vi "Dispose.vi"(8 "error in (no error)":errorcluster, 11 "BombedMazeGame":refnum<class "BombedMazeGame.lvclass">) -> (0 "error out":errorcluster)   [LabVIEW 2020, in "FactoryMethod.lvlib" / "NoParametrizedFactoryMethod.lvlib" / "BombedMazeGame.lvclass"]
uses:
  BombedMazeGame.lvclass
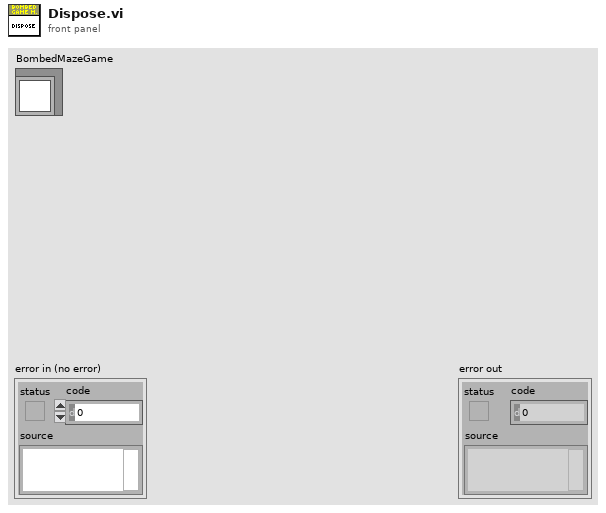
[diagram p1: front panel]
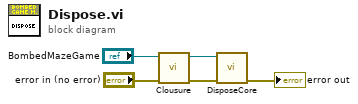
[diagram p0: block diagram]
diagram:
  n1 = call-dynamic "Clousure.vi"("error in (no error)"="error in (no error)", "BombedMazeGame"="BombedMazeGame") -> ("error out"=w1:errorcluster, "BombedMazeGame"=w2:refnum<class "BombedMazeGame.lvclass">)  [unwired: 8 in]
  n2 = call-dynamic "DisposeCore.vi"("error in (no error)"=w1, "BombedMazeGame"=w2) -> ("error out"=→"error out":errorcluster)  [unwired: 8 in, 1 out]
